vi "Read DebuggingTerminal.vi"(11 "Connection in":refnum<class "Connection.lvclass">) -> (2 "DebuggingTerminal":refnum<class "DebuggingTerminal.lvclass">, 3 "Connection out":refnum<class "Connection.lvclass">)   [LabVIEW 2013, in "MQTT_Connection.lvlib" / "Connection.lvclass"]
uses:
  Connection.lvclass
  MQTT_Base/DebuggingTerminal/DebuggingTerminal.lvclass
  Connection.lvclass/Connection.ctl
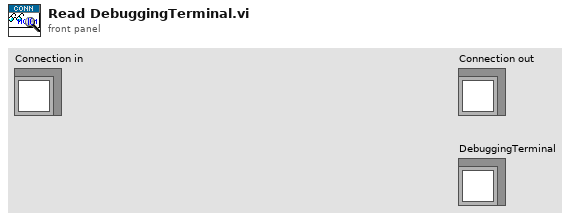
[diagram p1: front panel]
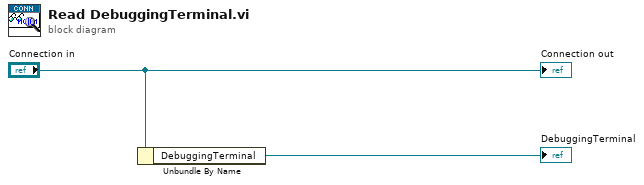
[diagram p0: block diagram]
diagram:
  n1 = Unbundle By Name("Connection in") -> ("DebuggingTerminal"=→"DebuggingTerminal":refnum<class "DebuggingTerminal.lvclass">)
  "Connection out" <- "Connection in"
